vi "Arm2Execute_CtrlOnly_ALT.vi"(8 "ReverseLimitSwitch":bool, 9 "ForwardLimitSwitch":bool, 10 "SensorVel Deg/Sec":dbl, 11 "SensorPos Deg":dbl) -> (1 "OnTarget":bool, 2 "Arm Demand Deg":dbl, 3 "Motor Output":dbl)   [LabVIEW 2023]
doc: "Arm Execute for 2024 robot"
uses:
  <vilib>/Rock Robotics/WPI/ThirdParty/JAS_Junk/TrajLib/Enum/DCMOTOR_TYPES_ENUM.ctl
  <vilib>/Rock Robotics/WPI/ThirdParty/JAS_Junk/TrajLib/VI/numCmd_ObtainQueue_OneDbl.vi
  <vilib>/Rock Robotics/WPI/ThirdParty/JAS_Junk/TrajLib/Trajectory_Library.lvlib
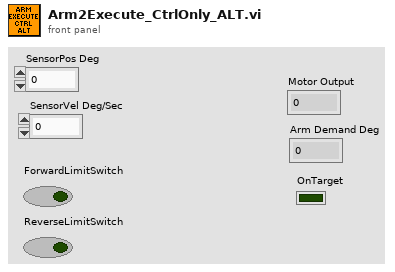
[diagram p1: front panel]
types:
  T1 = typedef "Trajectory_Library.lvlib/DCMOTOR_TYPES_ENUM.ctl" = enum16{"CIM", "AndyMark 9015", "Andy Mark RS 775 125", "Bag", "BaneBots RS 550", "BaneBots RS 775", "Falcon 500", "Mini CIM", "NEO", "NEO 550", "Romi BuiltIn", "Vex 775 Pro", "Snow Blower AM 2235A", "Bosch Seat AM 3493"}
  T2 = typedef "Trajectory_Library.lvlib/PosCtrl_Tuning_Type.ctl" = cluster{"Slope":dbl, "Offset":dbl, "Error Deadband":dbl, "At Reference Count":i32, "Negate Output":bool, "Max Allowd Position":dbl, "Min Allowd Position":dbl}
  T3 = typedef "Trajectory_Library.lvlib/LINEAR_SYSTEM_ID_SINGLE_JOINT_ARM_MODEL.ctl" = cluster{"DCMOTOR_TYPES":T1, "Num Motors":i32, "ArmLength_M":dbl, "massKg":dbl, "Gearing":dbl, "MOI kgm2":dbl, "Estimate MOI":bool}
  T4 = typedef "Trajectory_Library.lvlib/LINEAR_SYSTEM_LOOP_SNGJNTARM_CTRL_PARAMS.ctl" = cluster{"Ang Model Std Dev Rad":dbl, "Ang Meas Std Dev Rad":dbl, "Ang Ctrl Tol Rad":dbl, "Max Ctrl Out V":dbl, "Vel Model Std Dev Rad/Sec":dbl, "Vel Ctrl Tol Rad/Sec":dbl}
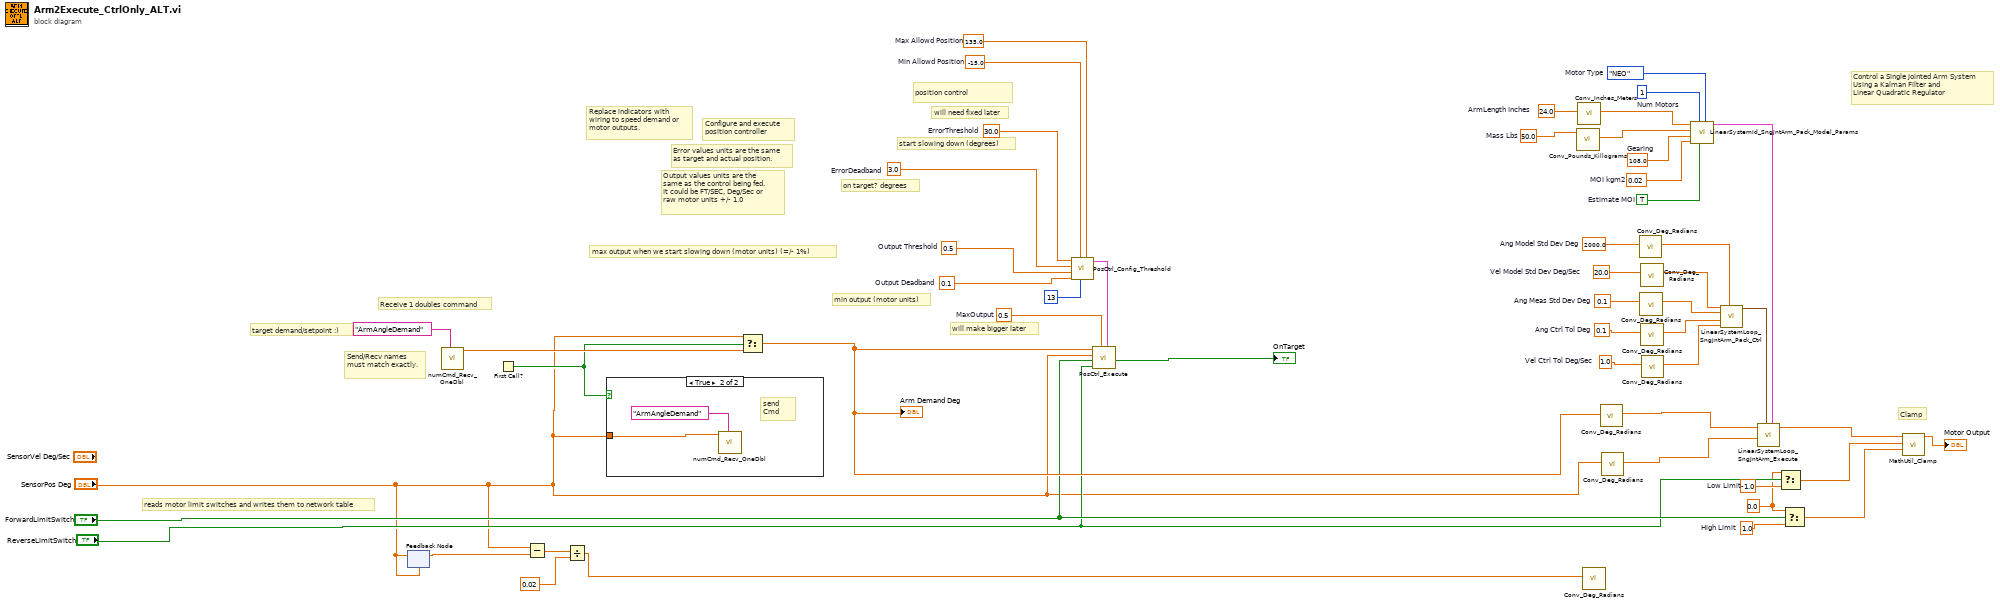
[diagram p0: block diagram]
diagram:
  w8 = 0.0 ("t")
  w32 = TRUE  # Estimate MOI
  w33 = 0.02  # MOI kgm2
  w29 = 24.0  # ArmLength Inches
  w34 = 108.0  # Gearing
  w30 = 50.0  # Mass Lbs
  w35 = 1  # Num Motors
  w36 = DCMOTOR_TYPES_ENUM."NEO"  # Motor Type
  w25 = 20.0  # Vel Model Std Dev Deg/Sec
  w24 = 0.1  # Ang Meas Std Dev Deg
  w23 = 0.1  # Ang Ctrl Tol Deg
  w22 = 1.0  # Vel Ctrl Tol Deg/Sec
  w26 = 2000.0  # Ang Model Std Dev Deg
  w11 = 1.0  # High Limit
  w12 = -1.0  # Low Limit
  w39 = 135.0  # Max Allowd Position
  w40 = -15.0  # Min Allowd Position
  w51 = 0.5  # MaxOutput
  w49 = 30.0  # ErrorThreshold
  w48 = 3.0  # ErrorDeadband
  w47 = 0.5  # Output Threshold
  w46 = 0.1  # Output Deadband
  # "Control a Single Jointed Arm System\nUsing a Kalman Filter and \nLinear Quadratic Regulator"
  # "Clamp"
  # "min output (motor units)"
  # "max output when we start slowing down (motor units) (=/- 1%)"
  # "on target? degrees"
  # "start slowing down (degrees)"
  # "will make bigger later"
  # "target demand/setpoint :)"
  # "Send/Recv names\nmust match exactly."
  # "Receive 1 doubles command"
  # "position control"
  # "will need fixed later"
  # "reads motor limit switches and writes them to network table"
  # "Replace indicators with\nwiring to speed demand or\nmotor outputs."
  # "Output values units are the\nsame as the control being fed.  \nIt could be FT/SEC, Deg/Sec or\nraw motor units +/- 1.0"
  # "Error values units are the same \nas target and actual position."
  # "Configure and execute \nposition controller"
  n1 = feedback-in #1("SensorPos Deg") -> ()
  n2 = feedback #1("SensorPos Deg") -> (w4:dbl)
  n3 = call <vilib>:"numCmd_Recv_OneDbl.vi"("Command Name"="ArmAngleDemand") -> ("Value"=w44:dbl)  [unwired: 8 in, 2 out]
  n4 = First Call?() -> (First Call?: T/F=w43:bool)
  n5 = Subtract(x="SensorPos Deg", y=w4) -> (x-y=w3:dbl)
  n6 = Divide(x=w3, y=0.02) -> (x/y=w1:dbl)
  n7 = case shown="True" w43 {
    tunnel: "SensorPos Deg" -> [_ w52]
    frame False {
    }
    frame True {
      # "send\nCmd"
      n8 = call <vilib>:"numCmd_Recv_OneDbl.vi"("Command Name"="ArmAngleDemand", "Initial Value"=w52) -> ()  [unwired: 7 in, 3 out]
    }
  }
  n9 = Select(t="SensorPos Deg", s=w43, f=w44) -> (s? t:f=w14:dbl)
  "Arm Demand Deg" <- w14
  n10 = call <vilib>:"PosCtrl_Config_Threshold.vi"("Max Allowd Position"=w39, "At Reference Count"=13, "Min Allowd Position"=w40, "Output Deadband"=w46, "Output Threshold"=w47, "ErrorDeadband"=w48, "ErrorThreshold"=w49) -> ("PosCtrl_Config_Params"=w50:T2)  [unwired: 4 in]
  n11 = call <vilib>:"PosCtrl_Execute.vi"("PosCtrl_Config_Params"=w50, "MaxOutput"=w51, "Rev Limit Switch"="ReverseLimitSwitch", "Fwd Limit Switch"="ForwardLimitSwitch", "CurrentPosition"="SensorPos Deg", "TargetPosition"=w14) -> ("OnTarget"=→"OnTarget":bool)  [unwired: 3 in, 2 out]
  n12 = call <vilib>:"Conv_Pounds_Killograms.vi"("Pounds"=w30) -> ("Killograms"=w31:dbl)  [unwired: 10 in]
  n13 = call <vilib>:"Conv_Inches_Meters.vi"("INCH"=w29) -> ("Meters"=w28:dbl)  [unwired: 10 in]
  n14 = call <vilib>:"Conv_Deg_Radians.vi"("Degress"=w1) -> ()  [unwired: 10 in, 1 out]
  n15 = call <vilib>:"Conv_Deg_Radians.vi"("Degress"=w14) -> ("Radians"=w15:dbl)  [unwired: 10 in]
  n16 = call <vilib>:"Conv_Deg_Radians.vi"("Degress"="SensorPos Deg") -> ("Radians"=w13:dbl)  [unwired: 10 in]
  n17 = call <vilib>:"Conv_Deg_Radians.vi"("Degress"=w26) -> ("Radians"=w21:dbl)  [unwired: 10 in]
  n18 = call <vilib>:"Conv_Deg_Radians.vi"("Degress"=w24) -> ("Radians"=w19:dbl)  [unwired: 10 in]
  n19 = call <vilib>:"Conv_Deg_Radians.vi"("Degress"=w25) -> ("Radians"=w20:dbl)  [unwired: 10 in]
  n20 = call <vilib>:"Conv_Deg_Radians.vi"("Degress"=w23) -> ("Radians"=w18:dbl)  [unwired: 10 in]
  n21 = call <vilib>:"Conv_Deg_Radians.vi"("Degress"=w22) -> ("Radians"=w17:dbl)  [unwired: 10 in]
  n22 = call <vilib>:"LinearSystemId_SngJntArm_Pack_Model_Params.vi"("DCMOTOR_TYPES"=w36, "Estimate MOI"=w32, "Num Motors"=w35, "MOI kgm2"=w33, "Gearing"=w34, "massKg"=w31, "ArmLength_M"=w28) -> ("SngJntArmSim_Model _Params"=w27:T3)  [unwired: 4 in]
  n23 = call <vilib>:"LinearSystemLoop_SngJntArm_Pack_Ctrl.vi"("Ang Model Std Dev Rad"=w21, "Vel Ctrl Tol Rad/Sec"=w17, "Ang Ctrl Tol Rad"=w18, "Ang Meas Std Dev Rad"=w19, "Vel Model Std Dev Rad/Sec"=w20) -> ("LinearSystemLoop_SngJntArm_Ctrl_Params"=w37:T4)  [unwired: 6 in]
  n24 = call <vilib>:"LinearSystemLoop_SngJntArm_Execute.vi"("LinearSystem_ID_SngJntArm_Model"=w27, "LinearSystem_SngJntArm_Ctrl_Params"=w37, "Process Variable\nRadians"=w13, "Ang Pos SP Rad"=w15) -> ("Motor Dmd"=w16:dbl)  [unwired: 3 in, 4 out]
  n25 = Select(t=w8, s="ReverseLimitSwitch", f=w12) -> (s? t:f=w7:dbl)
  n26 = Select(t=w8, s="ForwardLimitSwitch", f=w11) -> (s? t:f=w6:dbl)
  n27 = call <vilib>:"MathUtil_Clamp.vi"("High Limit"=w6, "Low Limit"=w7, "Value"=w16) -> ("Result"=→"Motor Output":dbl)  [unwired: 8 in]
